vi "test.vi"() -> ()   [LabVIEW 2009, in "CS POLARIS BME DG Client.lvlib"]
uses:
  CS POLARIS BME DG Client.lvlib
panel:
  in  "Numeric":dbl
  in  "stop":bool
  in  "ms":i32
  in  "µs":i32 min=-1000 max=1000
  in  "ns":i32 min=-1000 max=1000
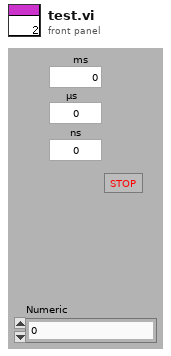
[diagram p1: front panel]
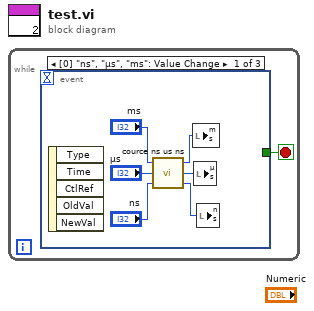
[diagram p0: block diagram]
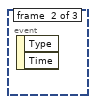
[diagram p2: hidden frame]
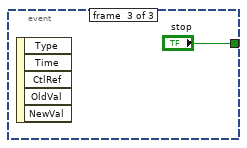
[diagram p3: hidden frame]
diagram:
  n1 = while {
    stop <- w1 stop-if-true
    n2 = event shown="[0] \"ns\", \"µs\", \"ms\": Value Change" {
      selector: _ -> [_ _ _]
      dyn-events: _ -> [_ _ _]
      timeout: _ -> [_ _ _]
      tunnel: [_ _ "stop"] -> w1
      event #0 {
        n3 = event-data() -> ()  [unwired: 1 in, 5 out]
        n4 = call "cource ns us ns.vi"("ns"="ns", "µs"="µs", "ms"="ms") -> ("ns out"=w2:i32, "µs out"=w3:i32, "ms out"=w4:i32)
        n5 = local write "ms"(w4) -> ()
        n6 = local write "µs"(w3) -> ()
        n7 = local write "ns"(w2) -> ()
      }
      event #1 {
        n8 = event-data() -> ()  [unwired: 1 in, 2 out]
      }
      event #2 {
        n9 = event-data() -> ()  [unwired: 1 in, 5 out]
      }
    }
  }
